vi "GEA3 HEWH Mixing Valve.vi"(8 "Error In":errorcluster, 10 "ERD Data In":T1[](array[typedef]) {"ERD Number" format="%.0x"}, 11 "GEA3 ERD Data":T2) -> (0 "Error Out":errorcluster, 2 "ERD Data Out":T1[](array[typedef]) {"ERD Number" format="%.0x"}, 3 "GEA3 ERD Data Out":T2, 5 "Mix Valve Data":string[][](array[string]))   [LabVIEW 2023]
uses:
  type defs/ERD Read Data Out.ctl
  Type Definitions/GEA3 HEWH ERD Data.ctl
  Type Definitions/GEA3 HEWH Mixing Valve.ctl
  library/GEA2_Toolkit.lvlib
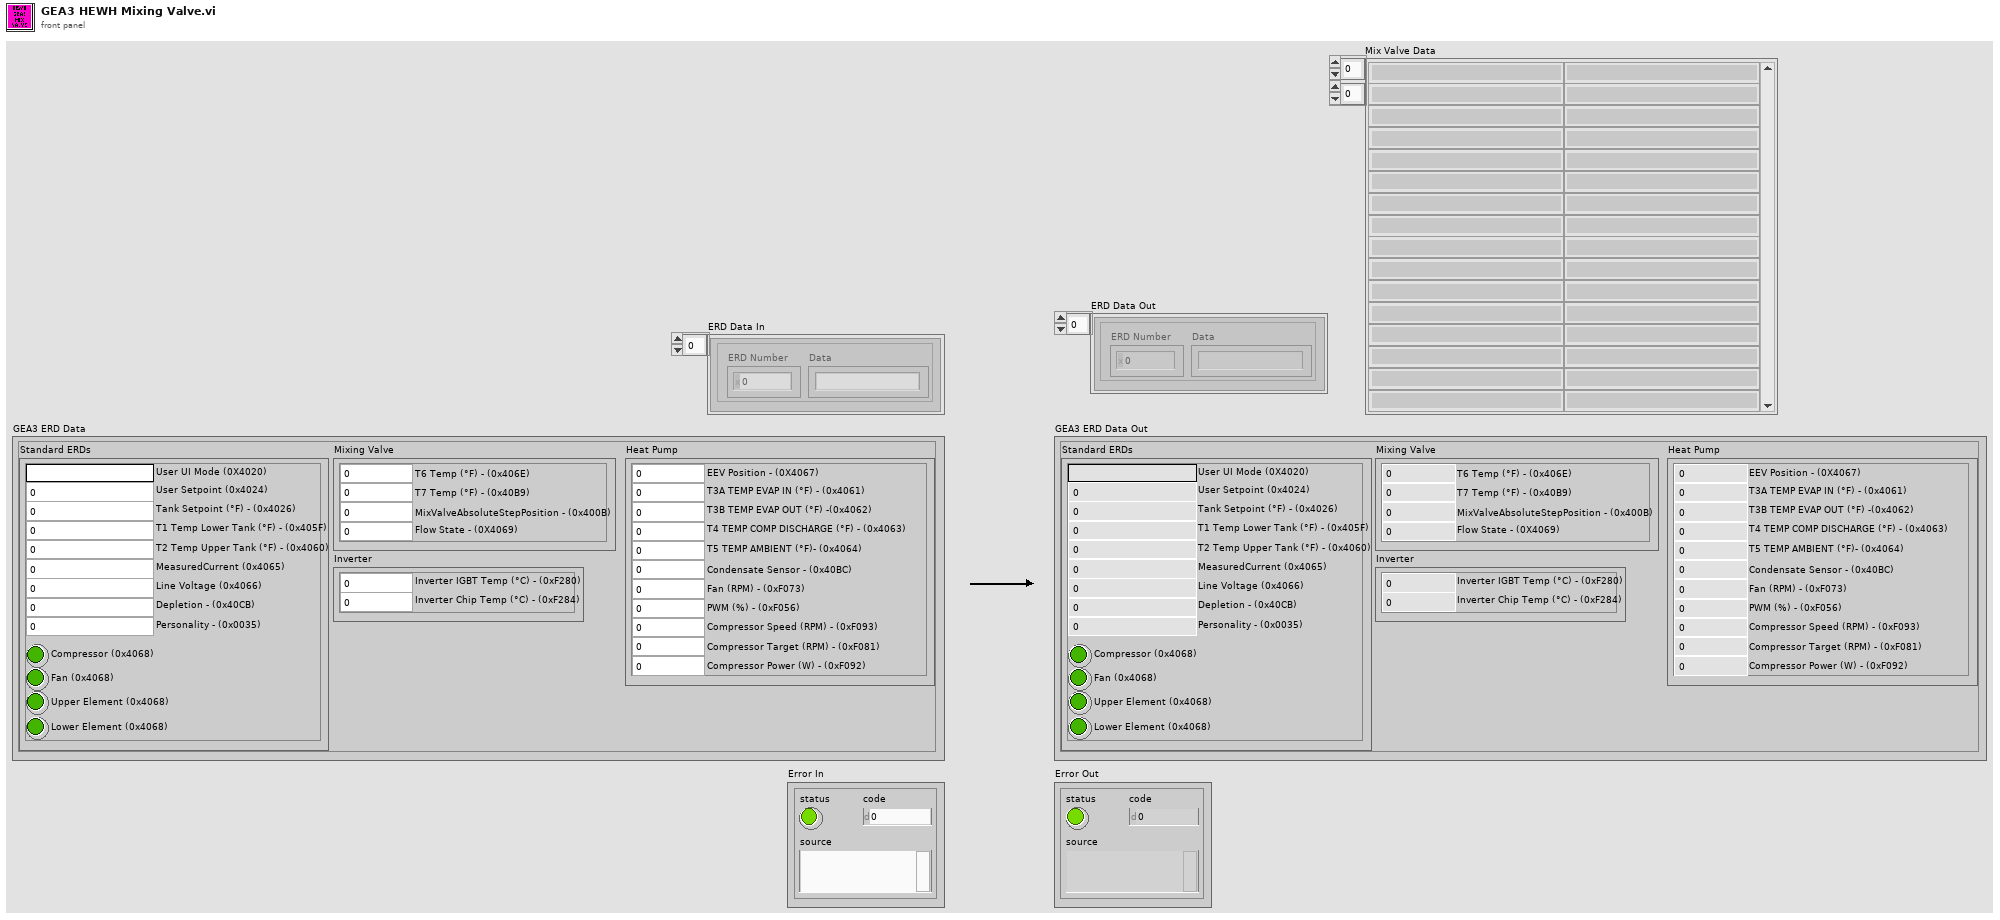
[diagram p1: front panel]
types:
  T1 = typedef "GEA2_Toolkit.lvlib/ERD Read Data Out.ctl" = cluster{"ERD Number":u16, "Data":string}
  T2 = typedef "GEA3 HEWH ERD Data.ctl" = cluster{"Mixing Valve":T3, "Standard ERDs":cluster{"User UI Mode (0X4020)":string, "User Setpoint (0x4024)":u16, "Compressor (0x4068)":bool, "Lower Element (0x4068)":bool, "Upper Element (0x4068)":bool, "Fan (0x4068)":bool, "T1 Temp Lower Tank (°F) - (0x405F)":dbl, "T2 Temp Upper Tank (°F) - (0x4060)":dbl, "Line Voltage (0x4066)":u16, "MeasuredCurrent (0x4065)":dbl, "Tank Setpoint (°F) - (0x4026)":u16, "Depletion - (0x40CB)":u16, "Personality - (0x0035)":u16}, "Heat Pump":cluster{"EEV Position - (0X4067)":u16, "T3A TEMP EVAP IN (°F) - (0x4061)":dbl, "T3B TEMP EVAP OUT (°F) -(0x4062)":dbl, "T4 TEMP COMP DISCHARGE (°F) - (0x4063)":dbl, "T5 TEMP AMBIENT (°F)- (0x4064)":dbl, "Condensate Sensor - (0x40BC)":u16, "Fan (RPM) - (0xF073)":u16, "PWM (%) - (0xF056)":u16, "Compressor Speed (RPM) - (0xF093)":u16, "Compressor Target (RPM) - (0xF081)":u16, "Compressor Power (W) - (0xF092)":u16}, "Inverter":cluster{"Inverter IGBT Temp (°C) - (0xF280)":dbl, "Inverter Chip Temp (°C) - (0xF284)":dbl}}
  T3 = typedef "GEA3 HEWH Mixing Valve.ctl" = cluster{"T7 Temp (°F) - (0x40B9)":dbl, "MixValveAbsoluteStepPosition - (0x400B)":i16, "Flow State - (0X4069)":u8, "T6 Temp (°F) - (0x406E)":dbl}
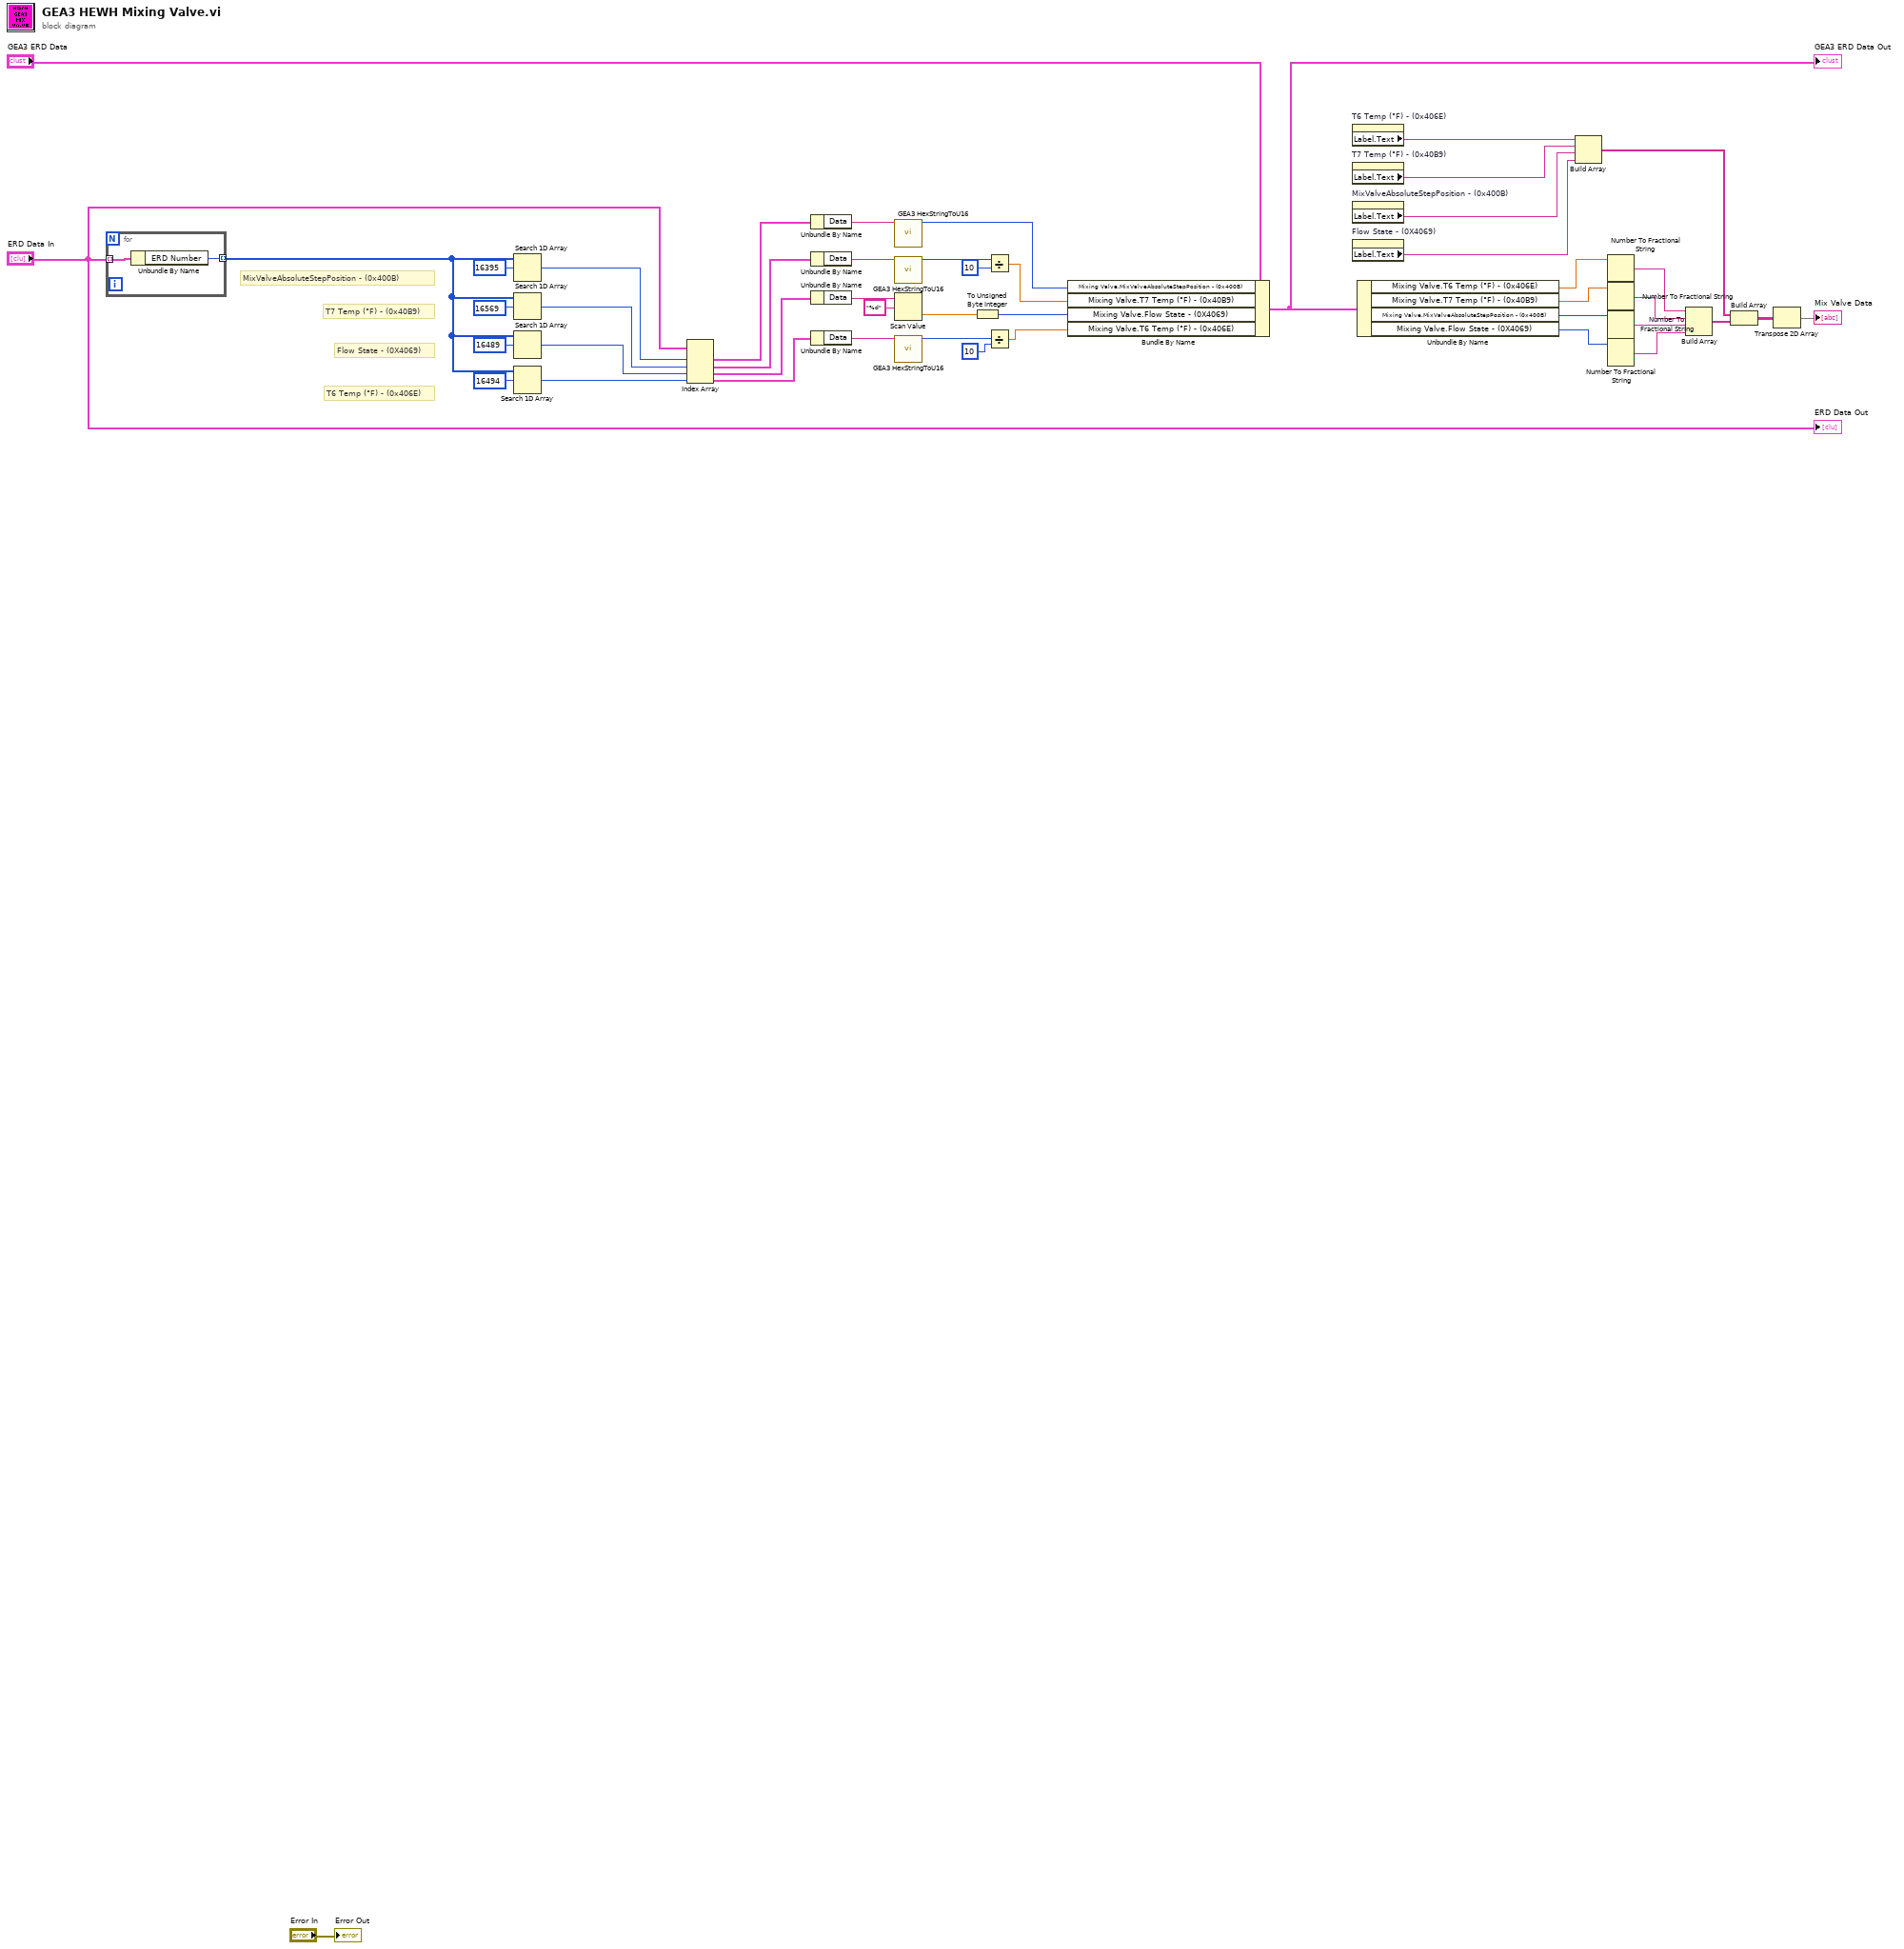
[diagram p0: block diagram]
diagram:
  # "Flow State - (0X4069)"
  # "MixValveAbsoluteStepPosition - (0x400B)"
  # "T7 Temp (°F) - (0x40B9)"
  # "T6 Temp (°F) - (0x406E)"
  n1 = for {
    tunnel: "ERD Data In" -> [w49] mode=indexing
    tunnel: [w48] -> w10 mode=indexing
    n2 = Unbundle By Name(w49) -> ("ERD Number"=w48:u16)
  }
  n3 = Search 1D Array(1D array=w10, element=u16 16395 ("ERD Number")) -> (index of element=w31:i32)  [unwired: 1 in]
  n4 = Search 1D Array(1D array=w10, element=u16 16569 ("ERD Number")) -> (index of element=w30:i32)  [unwired: 1 in]
  n5 = Search 1D Array(1D array=w10, element=u16 16489 ("ERD Number")) -> (index of element=w12:i32)  [unwired: 1 in]
  n6 = Search 1D Array(1D array=w10, element=u16 16494 ("ERD Number")) -> (index of element=w8:i32)  [unwired: 1 in]
  n7 = Index Array(array="ERD Data In", index #1=w31, index #2=w30, index #3=w12, index #4=w8) -> (element #1=w17:T1, element #2=w16:T1, element #3=w11:T1, element #4=w7:T1)
  n8 = Unbundle By Name(w17) -> ("Data"=w45:string)
  n9 = Unbundle By Name(w16) -> ("Data"=w41:string)
  n10 = Unbundle By Name(w11) -> ("Data"=w37:string)
  n11 = Unbundle By Name(w7) -> ("Data"=w29:string)
  n12 = call "GEA3 HexStringToU16.vi"("Input String"=w45) -> ("Number Out"=w44:u16)  [unwired: 14 in]
  n13 = call "GEA3 HexStringToU16.vi"("Input String"=w41) -> ("Number Out"=w43:u16)  [unwired: 14 in]
  n14 = Scan Value(string=w37, format string="%d") -> (value=w39:dbl)  [unwired: 1 in, 1 out]
  n15 = call "GEA3 HexStringToU16.vi"("Input String"=w29) -> ("Number Out"=w27:u16)  [unwired: 14 in]
  n16 = To Unsigned Byte Integer(number=w39) -> (unsigned 8bit integer=w15:u8)
  n17 = Divide(x=w43, y=u16 10) -> (x/y=w40:dbl)
  n18 = Divide(x=w27, y=u16 10) -> (x/y=w26:dbl)
  n19 = Bundle By Name(cluster="GEA3 ERD Data", "Mixing Valve.MixValveAbsoluteStepPosition - (0x400B)"=w44, "Mixing Valve.T7 Temp (°F) - (0x40B9)"=w40, "Mixing Valve.Flow State - (0X4069)"=w15, "Mixing Valve.T6 Temp (°F) - (0x406E)"=w26) -> (w25:T2)
  "GEA3 ERD Data Out" <- w25
  n20 = property on="T6 Temp (°F) - (0x406E)" class="DigNum (strict)"() -> ("Label.Text"=w4:string)  [unwired: 2 in, 2 out]
  n21 = property on="T7 Temp (°F) - (0x40B9)" class="DigNum (strict)"() -> ("Label.Text"=w3:string)  [unwired: 2 in, 2 out]
  n22 = property on="MixValveAbsoluteStepPosition - (0x400B)" class="DigNum (strict)"() -> ("Label.Text"=w2:string)  [unwired: 2 in, 2 out]
  n23 = property on="Flow State - (0X4069)" class="DigNum (strict)"() -> ("Label.Text"=w1:string)  [unwired: 2 in, 2 out]
  n24 = Unbundle By Name(w25) -> ("Mixing Valve.T6 Temp (°F) - (0x406E)"=w6:dbl, "Mixing Valve.T7 Temp (°F) - (0x40B9)"=w24:dbl, "Mixing Valve.MixValveAbsoluteStepPosition - (0x400B)"=w22:i16, "Mixing Valve.Flow State - (0X4069)"=w13:u8)
  n25 = Build Array(w4, w3, w2, w1) -> (w21:string[])
  n26 = Number To Fractional String(number=w6) -> (F-format string=w5:string)  [unwired: 3 in]
  n27 = Number To Fractional String(number=w24) -> (F-format string=w23:string)  [unwired: 3 in]
  n28 = Number To Fractional String(number=w22) -> (F-format string=w14:string)  [unwired: 3 in]
  n29 = Number To Fractional String(number=w13) -> (F-format string=w9:string)  [unwired: 3 in]
  n30 = Build Array(w5, w23, w14, w9) -> (w18:string[])
  n31 = Build Array(w21, w18) -> (w20:string[][])
  n32 = Transpose 2D Array(2D array=w20) -> (transposed array=→"Mix Valve Data":string[][])
  "Error Out" <- "Error In"
  "ERD Data Out" <- "ERD Data In"
